vi "Get Array Value at Index - 1D Array String.vi"(8 "error in (no error)":errorcluster, 9 "Default Value if JSON Null":string[](array[string]), 10 "Index":i32, 11 "JSON Tree In (JSON Array)":variant) -> (0 "error out":errorcluster, 1 "is JSON Null?":bool, 2 "1D String Array Value":string[](array[string]), 3 "JSON Tree Out Passthrough":variant)   [LabVIEW 2011, in "i3-json.lvlib"]
doc: "Use this template to build a VI to use as a subVI."
uses:
  i3-json.lvlib
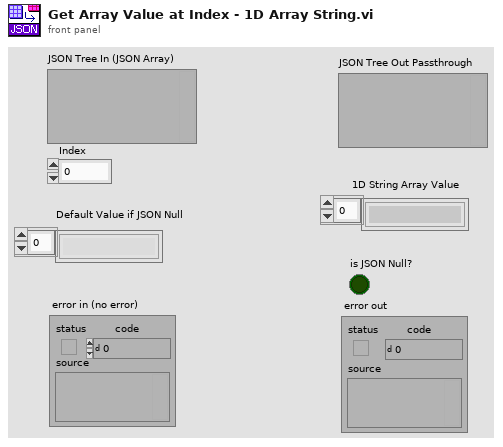
[diagram p1: front panel]
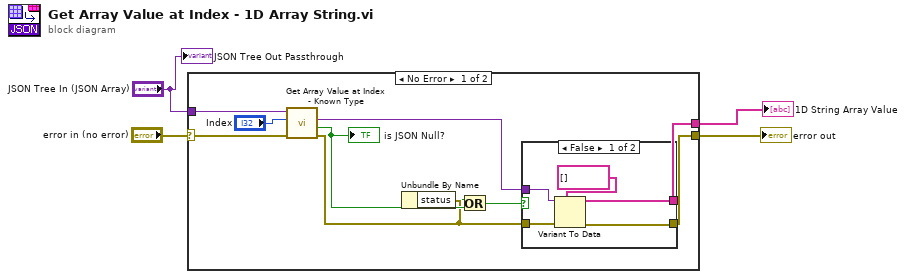
[diagram p0: block diagram]
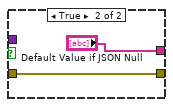
[diagram p2: hidden frame]
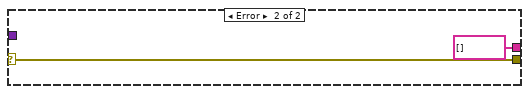
[diagram p3: hidden frame]
diagram:
  n1 = case shown="No Error" "error in (no error)" {
    selector: "error in (no error)" -> [w12 w23]
    tunnel: [w10 w23] -> w3
    tunnel: "JSON Tree In (JSON Array)" -> [w14 _]
    tunnel: [w7 string[] [] ("Default Value if JSON Null")] -> w2
    frame No Error {
      n2 = call "Get Array Value at Index - Known Type.vi"("error in (no error)"=w12, "Index"="Index", "JSON Tree In (JSON Array)"=w14) -> ("error out"=w6:errorcluster, "is JSON Null?"=w8:bool, "Value"=w9:variant)  [unwired: 3 in, 3 out]
      "is JSON Null?" <- w8
      n3 = Unbundle By Name(w6) -> ("status"=w5:bool)
      n4 = Or(x=w5, y=w8) -> (x .or. y?=w11:bool)
      n5 = case shown="False" w11 {
        tunnel: w6 -> [w19 w21]
        tunnel: [w16 w21] -> w10
        tunnel: w9 -> [w18 _]
        tunnel: [w17 "Default Value if JSON Null"] -> w7
        frame False {
          n6 = Variant To Data(error in=w19, type=string[] [], Variant=w18) -> (data=w17:string[], error out=w16:errorcluster)
        }
        frame True {
        }
      }
    }
    frame Error {
    }
  }
  "error out" <- w3
  "1D String Array Value" <- w2
  "JSON Tree Out Passthrough" <- "JSON Tree In (JSON Array)"
